vi "test.workspace_create_datasource_and_connection_in_incorrect_workspace.vi"   [LabVIEW 2020]
uses:
  730c9c5b-7bb2-47cf-818b-6e2ed47344d4.vi
  Nominal Client/Nominal Client.lvclass
  <vilib>/addons/_JKI Toolkits/Caraya/classes/Test/Test.lvclass
  <vilib>/addons/_JKI Toolkits/Caraya/classes/Assert/Assert.lvclass
  <vilib>/addons/_JKI Toolkits/Caraya/classes/Assert/Assert Not Error.vi
  02679ea1-62f9-4fe0-ba26-58395852097e.vi
  be3aaae4-45ad-4ded-8da6-0c8c22575439.vi
  <vilib>/addons/_JKI Toolkits/Caraya/classes/Assert/Assert Error.vi
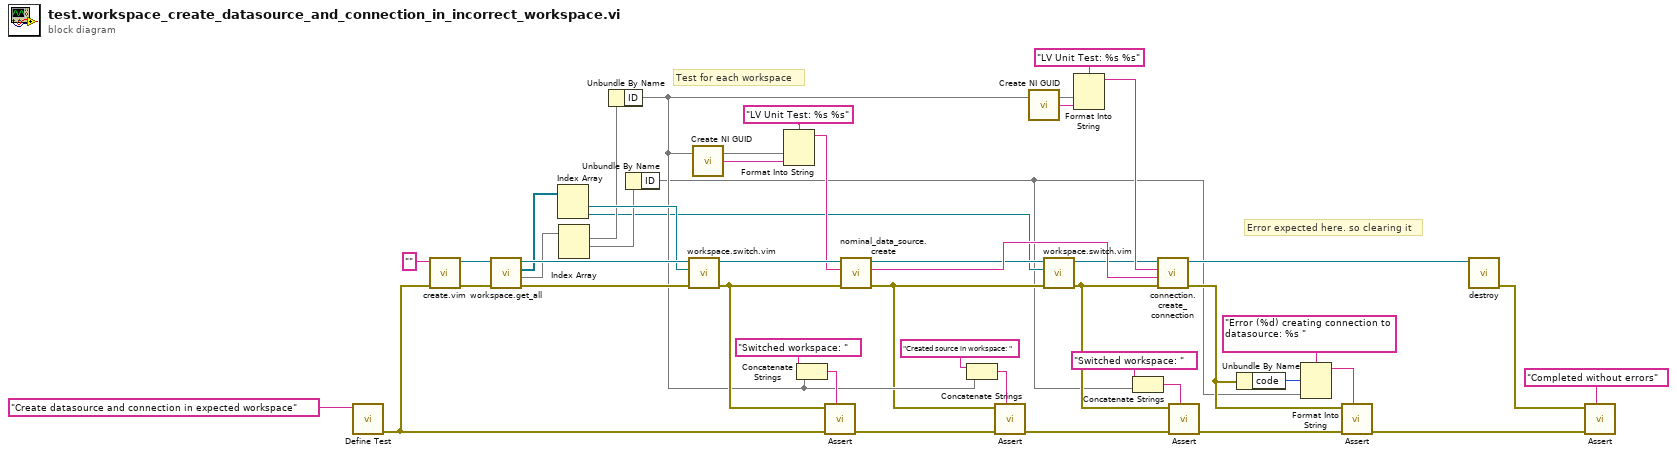
[diagram p0: block diagram]
diagram:
  # "Error expected here. so clearing it"
  # "Test for each workspace"
  n1 = call <vilib>:"Define Test.vi"("Label (VI Title)"="Create datasource and connection in expected workspace") -> ("error out"=w36:errorcluster)  [unwired: 9 in, 1 out]
  n2 = call "create.vim"("error in"=w36, "API Token (string or path)"="" ("Workspace RID (string or path)")) -> ("error out"=w42:errorcluster, "Nominal Client"=w43:refnum<class "Nominal Client.lvclass">)  [unwired: 7 in, 1 out]
  n3 = call "workspace.get_all.vi"("error in"=w42, "Nominal Client in"=w43) -> ("error out"=w37:errorcluster, 1:w17, "Workspaces"=w34:refnum<class "workspace.lvclass">[], "Nominal Client out"=w39:refnum<class "Nominal Client.lvclass">)  [unwired: 6 in]
  n4 = Index Array(array=w34) -> (element #1=w33:refnum<class "workspace.lvclass">, element #2=w6:refnum<class "workspace.lvclass">)  [unwired: 2 in]
  n5 = Index Array(array=w17) -> (element #1=w16, element #2=w11)  [unwired: 2 in]
  n6 = Unbundle By Name(w16) -> ("ID"=w18)
  n7 = Unbundle By Name(w11) -> ("ID"=w2)
  n8 = call "workspace.switch.vim"("error in"=w37, "Workspace (Object, RID, Path)"=w33, "Nominal Client in"=w39) -> ("error out"=w31:errorcluster, "Nominal Client out"=w32:refnum<class "Nominal Client.lvclass">)  [unwired: 7 in]
  n9 = call <vilib>:"Create NI GUID.vi"() -> ("NI GUID"=w29:string)
  n10 = Format Into String(format string="LV Unit Test: %s %s", w18, w29) -> (resulting string=w28:string)  [unwired: 2 in, 1 out]
  n11 = Concatenate Strings("Switched workspace: " ("Label"), w18) -> (w21:string)
  n12 = call-poly <vilib>:"Assert.vi"("Label"=w21, "error in (no error)"=w36, "Not Error?"=w31) -> ("error out"=w27:errorcluster)  [unwired: 7 in, 1 out]
  n13 = call "nominal_data_source.create.vi"("error in"=w31, "Name"=w28, "Nominal Client in"=w32) -> ("error out"=w14:errorcluster, "rid"=w26:string, "Nominal Client out"=w15:refnum<class "Nominal Client.lvclass">)  [unwired: 5 in, 1 out]
  n14 = Concatenate Strings("Created source in workspace: " ("Label"), w18) -> (w19:string)
  n15 = call-poly <vilib>:"Assert.vi"("Label"=w19, "error in (no error)"=w27, "Not Error?"=w14) -> ("error out"=w9:errorcluster)  [unwired: 7 in, 1 out]
  n16 = call <vilib>:"Create NI GUID.vi"() -> ("NI GUID"=w25:string)
  n17 = call "workspace.switch.vim"("error in"=w14, "Workspace (Object, RID, Path)"=w6, "Nominal Client in"=w15) -> ("error out"=w7:errorcluster, "Nominal Client out"=w10:refnum<class "Nominal Client.lvclass">)  [unwired: 7 in]
  n18 = Format Into String(format string="LV Unit Test: %s %s", w18, w25) -> (resulting string=w23:string)  [unwired: 2 in, 1 out]
  n19 = Concatenate Strings("Switched workspace: " ("Label"), w2) -> (w13:string)
  n20 = call "connection.create_connection.vi"("error in"=w7, "nominalDataSourceRid"=w26, "name"=w23, "Nominal Client in"=w10) -> ("error out"=w4:errorcluster, "Nominal Client out"=w38:refnum<class "Nominal Client.lvclass">)  [unwired: 4 in, 2 out]
  n21 = call-poly <vilib>:"Assert.vi"("Label"=w13, "error in (no error)"=w9, "Not Error?"=w7) -> ("error out"=w8:errorcluster)  [unwired: 7 in, 1 out]
  n22 = Unbundle By Name(w4) -> ("code"=w3:i32)
  n23 = Format Into String(format string="Error (%d) creating connection to datasource: %s " ("Label"), w3, w2) -> (resulting string=w1:string)  [unwired: 2 in, 1 out]
  n24 = call-poly <vilib>:"Assert.vi"("Label"=w1, "error in (no error)"=w8, "Error?"=w4) -> ("error out"=w35:errorcluster)  [unwired: 7 in, 1 out]
  n25 = call "destroy.vi"("Nominal Client"=w38) -> ("error out"=w41:errorcluster)  [unwired: 10 in]
  n26 = call-poly <vilib>:"Assert.vi"("Label"="Completed without errors", "error in (no error)"=w35, "Not Error?"=w41) -> ()  [unwired: 7 in, 2 out]
